vi "saveColumnHeaders.vi"(8 "error in (no error)":errorcluster, 11 "Logger in":refnum<class "Log.lvclass">) -> (0 "error out":errorcluster, 3 "Logger out":refnum<class "Log.lvclass">)   [LabVIEW 2013, in "Log.lvlib" / "Log.lvclass"]
uses:
  <userlib>/Common/Log/Log/Log.lvclass
  <userlib>/Common/Log/Log/Log.lvclass/Log.ctl
  <vilib>/Utility/file.llb/Write To Spreadsheet File (string).vi
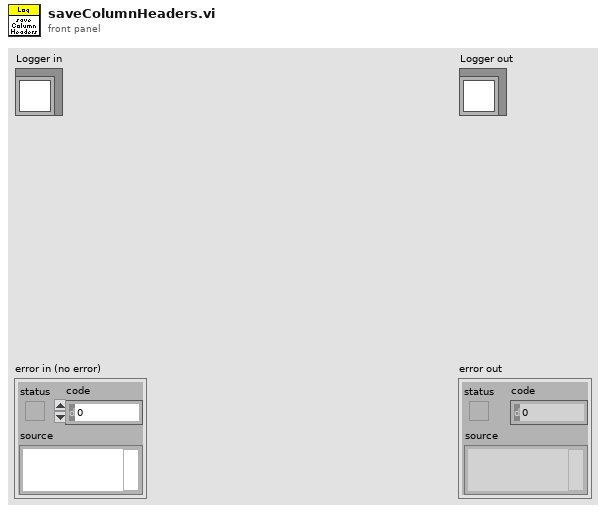
[diagram p1: front panel]
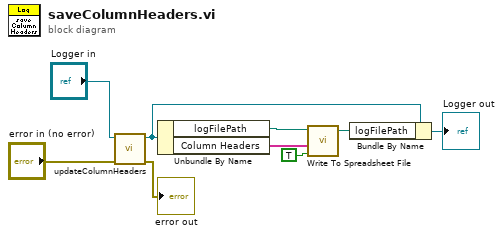
[diagram p0: block diagram]
diagram:
  n1 = call-dynamic "updateColumnHeaders.vi"("error in (no error)"="error in (no error)", "Logger in"="Logger in") -> ("error out"=→"error out":errorcluster, "Logger out"=w3:refnum<class "Log.lvclass">)  [unwired: 8 in]
  n2 = Unbundle By Name(w3) -> ("logFilePath"=w7:path, "Column Headers"=w5:string[])
  n3 = call-poly <vilib>:"Write To Spreadsheet File.vi"("append to file? (new file:F)"=TRUE, "1D data"=w5, "file path (dialog if empty)"=w7) -> ("new file path (Not A Path if cancelled)"=w8:path)  [unwired: 5 in]
  n4 = Bundle By Name(cluster=w3, "logFilePath"=w8) -> (→"Logger out":refnum<class "Log.lvclass">)
